vi "Parallel PID with I-zone (DBL).vi"(0 "setpoint":dbl format="%.2f", 1 "output range":cluster{"high":dbl, "low":dbl}={"high"=100.0, "low"=-100.0} {"low" format="%.2f"; "high" format="%.2f"}, 3 "alpha":dbl=nan format="%.2f", 5 "process variable":dbl format="%.2f", 7 "i-zone":dbl=-1.0 format="%.2f", 9 "PID gains":T1={"proportional gain (Kp)"=1.0, "integral time (Ki)"=0.0, "derivative time (Kd)"=0.0} {"derivative time (Kd)" format="%.3f"; "integral time (Ki)" format="%.3f"; "proportional gain (Kp)" format="%.3f"}, 11 "dt (s)":dbl=-1.0 format="%.3f", 12 "reinitialize? (F)":bool, 14 "FeedFwd Value":dbl format="%.2f") -> (4 "output":dbl format="%.2f", 6 "SP/PV Chart":cluster{"setpoint":dbl, "process variable":dbl}(graph), 10 "Err/Out Chart":cluster{dbl, dbl}(graph), 15 "dt out (s)":dbl format="%.3f")   [LabVIEW 2020]
doc: "Implements a parallel PID controller appropriate for robotics. The PID algorithm features control output range limiting with integrator anti-windup and bumpless controller output for PID gain changes. Include any feedforward amount that should be used to cancel constant forces or improve Velocity control."
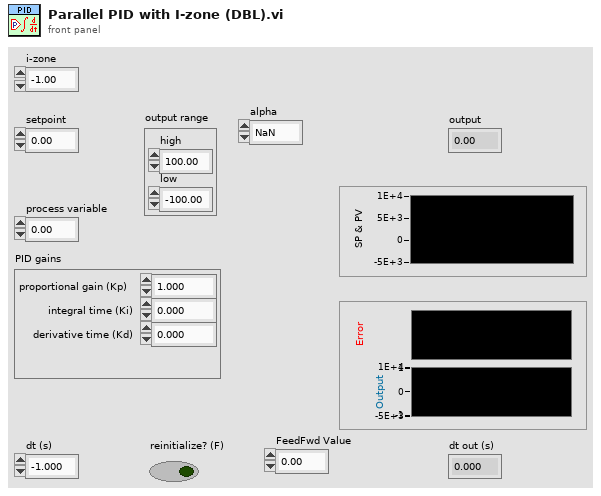
[diagram p1: front panel]
types:
  T1 = cluster{"proportional gain (Kp)":dbl, "integral time (Ki)":dbl, "derivative time (Kd)":dbl}
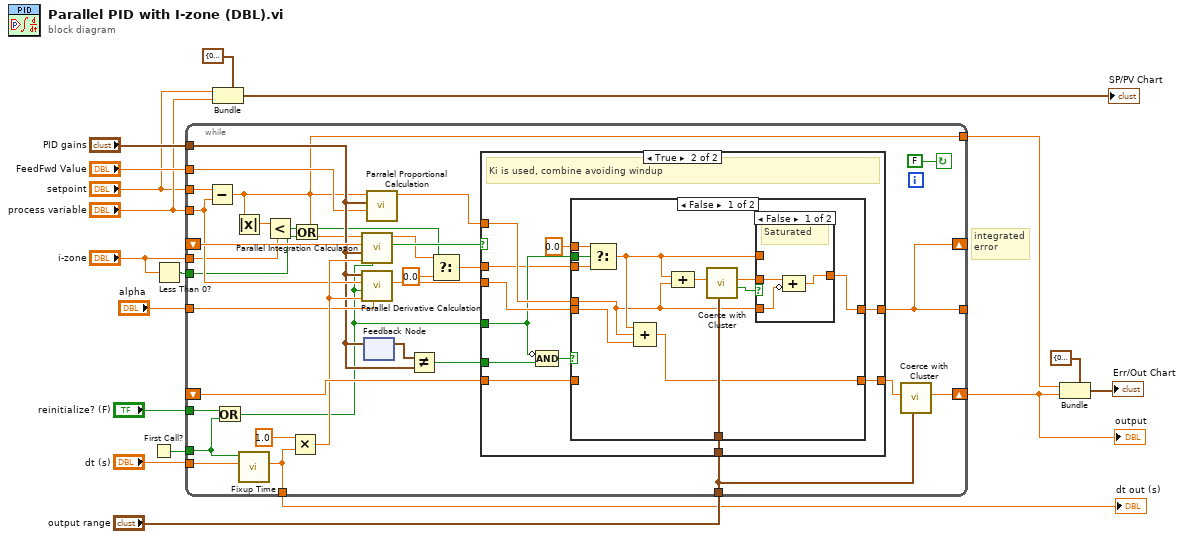
[diagram p0: block diagram]
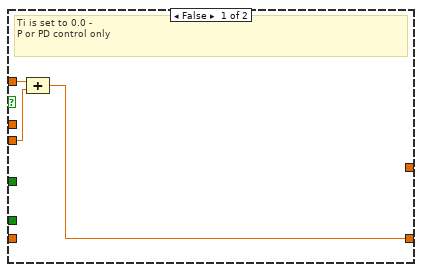
[diagram p2: hidden frame]
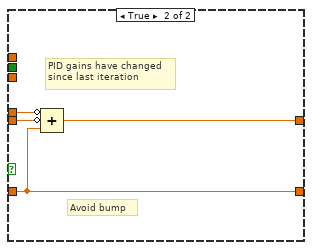
[diagram p4: hidden frame]
diagram:
  # "integrated\nerror"
  n1 = First Call?() -> (First Call?: T/F=w17:bool)
  n2 = Less Than 0?(x="i-zone") -> (x < 0?=w1:bool)
  n3 = while {
    tunnel: "dt (s)" -> [w48]
    tunnel: "process variable" -> [w39]
    shift-right: [w40] -> w5
    shift-left: _ -> [w50]
    shift-right: [w29] -> _
    shift-left: _ -> [w44]
    tunnel: w17 -> [w37]
    tunnel: "PID gains" -> [w32]
    tunnel: "output range" -> [w42]
    tunnel: [w45] -> w14
    tunnel: "FeedFwd Value" -> [w31]
    tunnel: "setpoint" -> [w38]
    tunnel: "reinitialize? (F)" -> [w36]
    tunnel: [w28] -> w4
    tunnel: "alpha" -> [w35]
    tunnel: [w29] -> _
    tunnel: "i-zone" -> [w26]
    tunnel: w1 -> [w20]
    stop <- FALSE continue-if-true
    n4 = Subtract(x=w38, y=w39) -> (x-y=w28:dbl)
    n5 = Or(x=w36, y=w37) -> (x .or. y?=w30:bool)
    n6 = Absolute Value(x=w28) -> (abs(x)=w27:dbl)
    n7 = call <vilib>:"Fixup Time.vi"("dt (s) in"=w48, "Initialize?:"=w37) -> ("dt (s) out"=w45:dbl)  [unwired: 9 in]
    n8 = Less?(x=w27, y=w26) -> (x < y?=w21:bool)
    n9 = Multiply(x=1.0 ("1/60"), y=w45) -> (x*y=w43:dbl)
    n10 = Or(x=w21, y=w20) -> (x .or. y?=w19:bool)
    n11 = call <vilib>:"Parallel Integration Calculation.vi"("Reinit"=w30, "dT"=w43, "PID gains"=w32, "Integration Error"=w44, "Curr Error"=w28) -> ("Integral Used"=w25:bool, "Integral Term"=w24:dbl)  [unwired: 5 in]
    n12 = call <vilib>:"Parallel Derivative Calculation.vi"("alpha"=w35, "dt"=w43, "Reinit"=w30, "process variable in"=w39, "PID gains"=w32) -> ("deriv Term"=w51:dbl)  [unwired: 6 in]
    n13 = feedback-in #1(w32) -> ()
    n14 = feedback #1() -> (w34:T1)  [unwired: 1 in]
    n15 = call <vilib>:"Parralel Proportional Calculation.vi"("FeedFwd Amount"=w31, "PID gains"=w32, "Error"=w28) -> ("Proportional Term"=w33:dbl)  [unwired: 8 in]
    n16 = Not Equal?(x=w34, y=w32) -> (x != y?=w47:bool)
    n17 = Select(t=w24, s=w19, f=0.0) -> (s? t:f=w22:dbl)
    n18 = case shown="True" w25 {
      tunnel: [_ w62] -> w29
      tunnel: w50 -> [_ w63]
      tunnel: w51 -> [w52 w61]
      tunnel: w30 -> [_ w60]
      tunnel: w47 -> [_ w59]
      tunnel: w42 -> [_ w58]
      tunnel: w22 -> [_ w57]
      tunnel: [w53 w56] -> w41
      tunnel: w33 -> [w54 w65]
      frame False {
        # "Ti is set to 0.0 -\nP or PD control only"
        n19 = Compound Arithmetic op=ADD(w54, w52) -> (w53:dbl)
      }
      frame True {
        # "Ki is used, combine avoiding windup"
        n20 = Compound Arithmetic op=AND(invert w60, w59) -> (w64:bool)
        n21 = case shown="False" w64 {
          tunnel: w57 -> [w75 _]
          tunnel: w65 -> [w67 w85]
          tunnel: w63 -> [_ w82]
          tunnel: w60 -> [w76 _]
          tunnel: [w77 w83] -> w62
          tunnel: w61 -> [w70 w84]
          tunnel: w58 -> [w71 _]
          tunnel: [w68 w82] -> w56
          tunnel: 0.0 -> [w66 _]
          frame False {
            n22 = Select(t=w66, s=w76, f=w75) -> (s? t:f=w69:dbl)
            n23 = Compound Arithmetic op=ADD(w69, w67, w70) -> (w68:dbl)
            n24 = Compound Arithmetic op=ADD(w69, w67) -> (w72:dbl)
            n25 = call <vilib>:"Coerce with Cluster.vi"("value in"=w72, "output range"=w71) -> ("coerced value"=w73:dbl, "In Range?"=w74:bool)  [unwired: 7 in]
            n26 = case shown="False" w74 {
              tunnel: w69 -> [_ w81]
              tunnel: [w78 w81] -> w77
              tunnel: w73 -> [w80 _]
              tunnel: w67 -> [w79 _]
              frame False {
                # "Saturated"
                n27 = Compound Arithmetic op=ADD(w80, invert w79) -> (w78:dbl)
              }
              frame True {
                # "! Saturated"
              }
            }
          }
          frame True {
            # "Avoid bump"
            # "PID gains have changed\nsince last iteration"
            n28 = Compound Arithmetic op=ADD(invert w85, invert w84, w82) -> (w83:dbl)
          }
        }
      }
    }
    n29 = call <vilib>:"Coerce with Cluster.vi"("value in"=w41, "output range"=w42) -> ("coerced value"=w40:dbl)  [unwired: 7 in, 1 out]
  }
  "output" <- w5
  "dt out (s)" <- w14
  n30 = Bundle(cluster=cluster{"setpoint":dbl, "process variable":dbl} {"setpoint"=0.0, "process variable"=0.0}, "setpoint"="setpoint", "process variable"="process variable") -> (→"SP/PV Chart":cluster{"setpoint":dbl, "process variable":dbl})
  n31 = Bundle(cluster=cluster{"Error":dbl, "Output":dbl} {"Error"=0.0, "Output"=0.0}, "Error"=w4, "Output"=w5) -> (→"Err/Out Chart":cluster{"Error":dbl, "Output":dbl})
